vi "Read Analysis ROI.vi"(8 "error in (no error)":errorcluster, 11 "Analysis Graph in":refnum<class "Analysis Graph.lvclass">) -> (0 "error out":errorcluster, 2 "ROI XYZ":T1, 3 "Analysis Graph out":refnum<class "Analysis Graph.lvclass">)   [LabVIEW 2023, in "Analysis Graph.lvclass"]
uses:
  Analysis Graph.lvclass
  Analysis Graph.lvclass/Analysis Graph.ctl
  Base Graph/Base Graph.lvclass
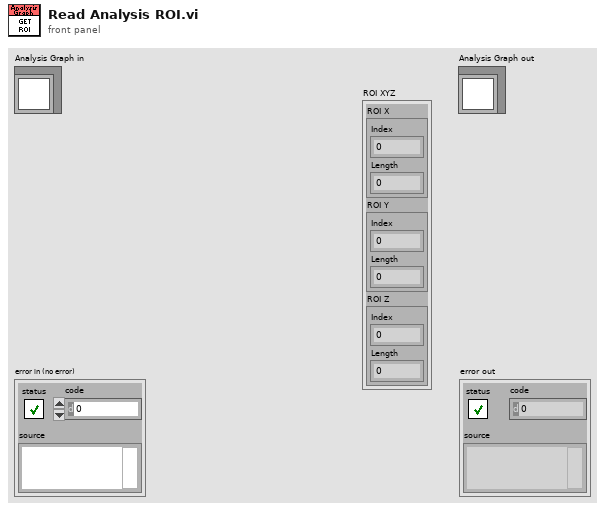
[diagram p1: front panel]
types:
  T1 = cluster{"ROI X":cluster{"Index":u32, "Length":u32}, "ROI Y":cluster{"Index":u32, "Length":u32}, "ROI Z":cluster{"Index":u32, "Length":u32}}
  T2 = cluster{"ROI X":cluster{"Index":u32, "Length":u32}, "ROI Y":cluster{"Index":u32, "Length":u32}}
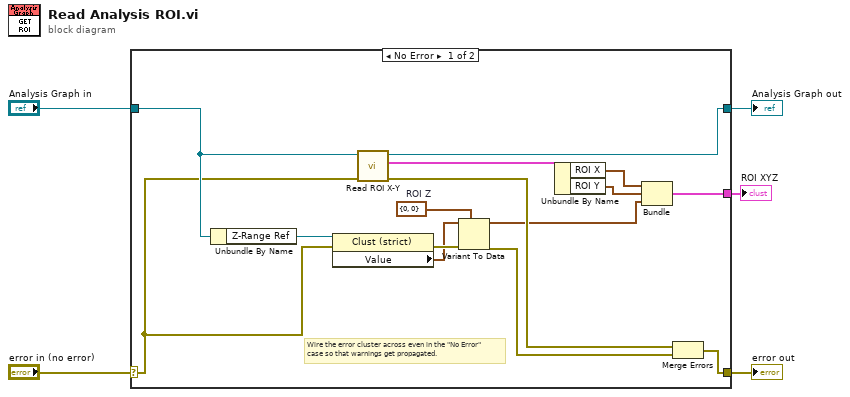
[diagram p0: block diagram]
diagram:
  n1 = case shown="No Error" "error in (no error)" {
    selector: "error in (no error)" -> [w18 w22]
    tunnel: [w16 w22] -> w4
    tunnel: [w17 w21] -> w2
    tunnel: "Analysis Graph in" -> [w19 w21]
    tunnel: [w14 _] -> w1
    frame No Error {
      w6 = cluster{"Index":u32, "Length":u32} {"Index"=0, "Length"=0}  # ROI Z
      # "Wire the error cluster across even in the \"No Error\"\ncase so that warnings get propagated."
      n2 = Unbundle By Name(w19) -> ("Z-Range Ref"=w20:refnum<vi>)
      n3 = property class="Clust (strict)"(reference=w20, error in=w18) -> (error out=w10:errorcluster, "Value"=w8:cluster{"Index":u32, "Length":u32})  [unwired: 1 out]
      n4 = call "Read ROI X-Y.vi"("error in (no error)"=w18, "Base Graph in"=w19) -> ("error out"=w15:errorcluster, "ROI XY"=w13:T2, "Base Graph out"=w17:refnum<class "Analysis Graph.lvclass">)  [unwired: 7 in]
      n5 = Variant To Data(error in=w10, type=w6, Variant=w8) -> (data=w7:cluster{"Index":u32, "Length":u32}, error out=w9:errorcluster)
      n6 = Unbundle By Name(w13) -> ("ROI X"=w12:cluster{"Index":u32, "Length":u32}, "ROI Y"=w11:cluster{"Index":u32, "Length":u32})
      n7 = Bundle("ROI X"=w12, "ROI Y"=w11, "ROI Z"=w7) -> (w14:T1)  [unwired: 1 in]
      n8 = Merge Errors(w15, w9) -> (w16:errorcluster)
    }
    frame Error {
    }
  }
  "error out" <- w4
  "Analysis Graph out" <- w2
  "ROI XYZ" <- w1
